vi "SmartMotor Read.vi"(0 "VISA resource IN":refnum<visa-resource-name>, 1 "Motor Number":i16, 2 "Read Command to Motor":string, 3 "Error In":errorcluster, 5 "Byte Count to Read":u32=1024) -> (4 "Return Buffer Count":u32, 6 "VISA resource OUT":refnum<visa-resource-name>, 7 "Motor Number OUT":i16, 8 "Response From Motor":string, 9 "Error Out":errorcluster)   [LabVIEW 2017, in "SmartMotor.lvclass"]
uses:
  SmartMotor.lvclass
  <vilib>/Instr/_visa.llb/VISA Flush IO Buffer Mask.ctl
panel:
  out "Complete Command Send":string
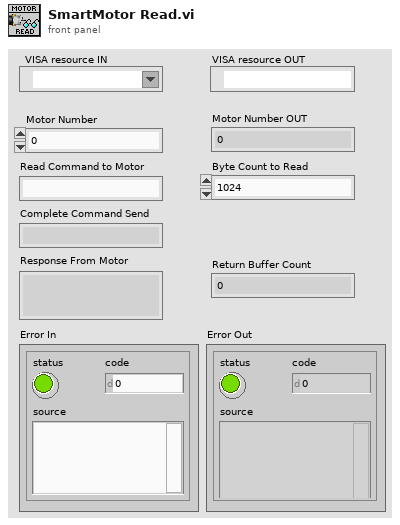
[diagram p1: front panel]
types:
  T1 = typedef "VISA Flush IO Buffer Mask.ctl" = u16
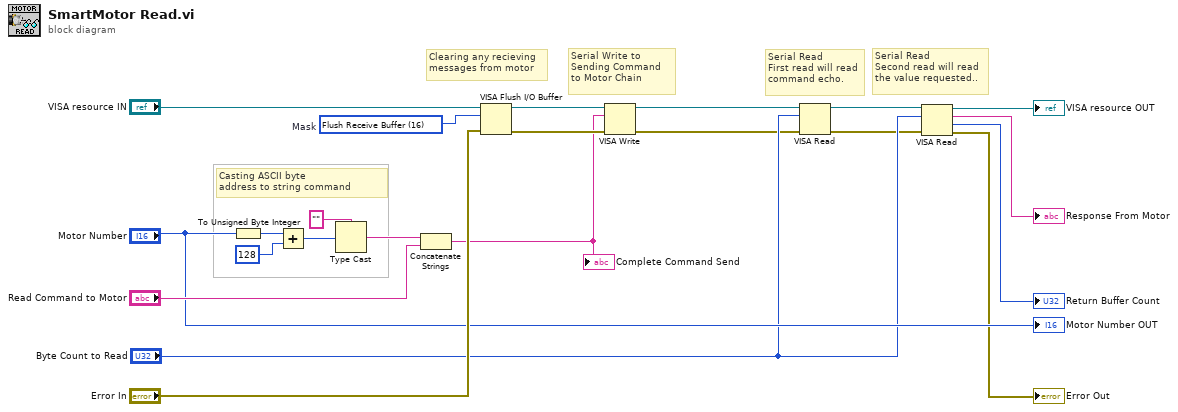
[diagram p0: block diagram]
diagram:
  w3 = T1 16 items=["Flush Receive Buffer"=16, "Write Transmit Buffer to Device"=32, "Flush Receive Buffer (No I/O)"=64, "Flush Transmit Buffer"=128]  # Mask
  # "Clearing any recieving\nmessages from motor"
  # "Serial Read\nSecond read will read\nthe value requested.."
  # "Serial Read\nFirst read will read\ncommand echo."
  # "Casting ASCII byte\naddress to string command"
  # "Serial Write to \nSending Command\nto Motor Chain"
  n1 = To Unsigned Byte Integer(number="Motor Number") -> (unsigned 8bit integer=w10:u8)
  n2 = Add(x=w10, y=u8 128) -> (x+y=w19:u8)
  n3 = Type Cast(type="", x=w19) -> (*(type *) &x=w20:string)
  n4 = Concatenate Strings(w20, "Read Command to Motor") -> (w4:string)
  "Complete Command Send" <- w4
  n5 = VISA Flush I/O Buffer(VISA resource name="VISA resource IN", mask (16)=w3, error in (no error)="Error In") -> (VISA resource name out=w12:refnum<visa-resource-name>, error out=w11:errorcluster)
  n6 = VISA Write(VISA resource name=w12, write buffer=w4, error in (no error)=w11) -> (VISA resource name out=w6:refnum<visa-resource-name>, error out=w2:errorcluster)  [unwired: 1 out]
  n7 = VISA Read(VISA resource name=w6, byte count="Byte Count to Read", error in (no error)=w2) -> (VISA resource name out=w7:refnum<visa-resource-name>, error out=w1:errorcluster)  [unwired: 2 out]
  n8 = VISA Read(VISA resource name=w7, byte count="Byte Count to Read", error in (no error)=w1) -> (VISA resource name out=→"VISA resource OUT":refnum<visa-resource-name>, read buffer=→"Response From Motor":string, return count=→"Return Buffer Count":u32, error out=→"Error Out":errorcluster)
  "Motor Number OUT" <- "Motor Number"
